vi "PH_Beckhoff_PPMA-Rods.set Digital Input GUI Elements.vi"(2 "Input Up GUI Refs":refnum<vi>[](array[refnum]), 3 "Input GUI Refs":T1, 4 "Digital Inputs":T2, 5 "error in":errorcluster) -> (19 "error out":errorcluster)   [LabVIEW 2014, in "PH_Beckhoff_PPMA-Rods.lvlib"]
doc: "This VI sets the digital Input GUI elements which is whether the rods ar up or not."
uses:
  PH_Beckhoff_PPMA-Rods.lvlib
  PH_Beckhoff/PH_Beckhoff.Digital Inputs.ctl
  PH_Beckhoff_PPMA-Rods.Rods Tags.ctl
  PH_Common/PH_Common.lvlib
  PH_Beckhoff/PH_Beckhoff.lvlib
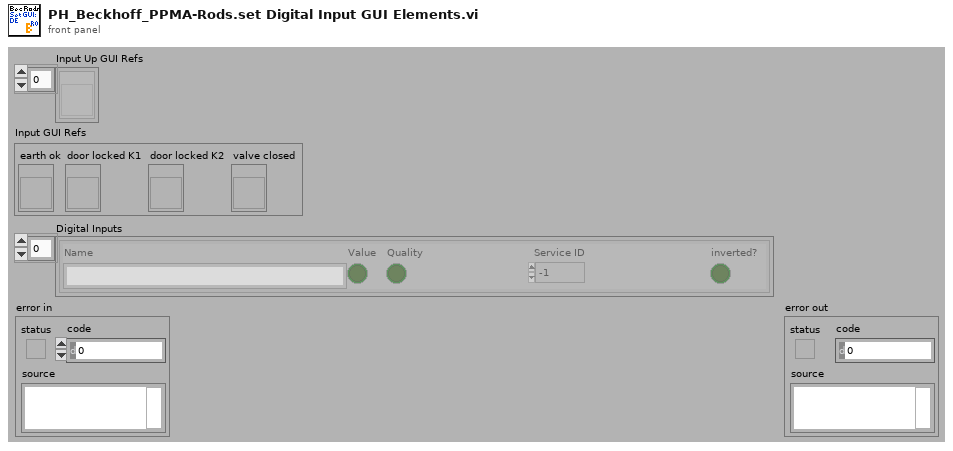
[diagram p1: front panel]
types:
  T1 = cluster{"earth ok":refnum<vi>, "door locked K1":refnum<vi>, "door locked K2":refnum<vi>, "valve closed":refnum<vi>}
  T2 = typedef "PH_Beckhoff.lvlib/PH_Beckhoff.Digital Inputs.ctl" = cluster{"Name":string, "Value":bool, "Quality":bool, "Service ID":i32, "inverted?":bool}[]
  T3 = typedef "PH_Beckhoff_PPMA-Rods.lvlib/PH_Beckhoff_PPMA-Rods.Rods Tags.ctl" = enum16{"Rod-up", "earth-ok", "door-locked-K1", "door-locked-K2", "watervalve-closed", "Rods-Chain-A-up", "Rods-Chain-B-up", "HV-Warnlamp-orange", "HV-Warnlamp-green", "Status-Rods-PU-1", "Status-Rods-PU-2", "Status-Rods-PU-3", "Status-Rods-PU-4", "Status-Rods-PU-5", "Status-Rods-PU-6", "Status-Rods-PU-7", "Status-Rods-PU-8", "Status-Rods-PU-9", "Status-Rods-PU-10", "Status-Rods-FR", "Status-Rods-PILC"}
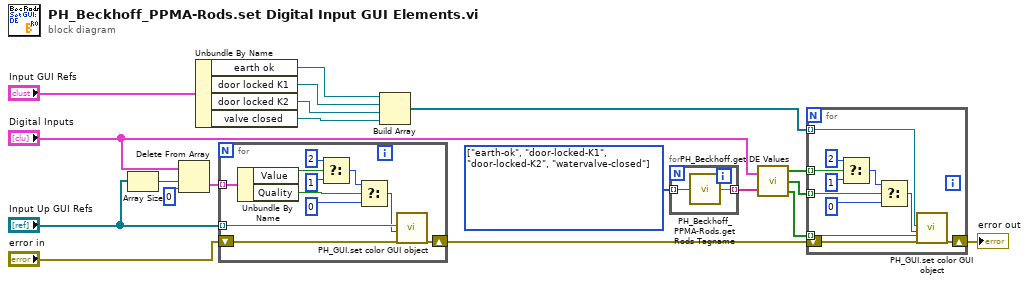
[diagram p0: block diagram]
diagram:
  w7 = T3[] [enum."earth-ok", enum."door-locked-K1", enum."door-locked-K2", enum."watervalve-closed"] items=["Rod-up", "earth-ok", "door-locked-K1", "door-locked-K2", "watervalve-closed", "Rods-Chain-A-up", "Rods-Chain-B-up", "HV-Warnlamp-orange", "HV-Warnlamp-green", "Status-Rods-PU-1", "Status-Rods-PU-2", "Status-Rods-PU-3", "Status-Rods-PU-4", "Status-Rods-PU-5", "Status-Rods-PU-6", "Status-Rods-PU-7", "Status-Rods-PU-8", "Status-Rods-PU-9", "Status-Rods-PU-10", "Status-Rods-FR", "Status-Rods-PILC"]
  n1 = Array Size(array="Input Up GUI Refs") -> (size(s)=w16:i32)
  n2 = Delete From Array(array="Digital Inputs", length=w16, index=0) -> (deleted portion=w1:T2)  [unwired: 1 out]
  n3 = Unbundle By Name("Input GUI Refs") -> ("earth ok"=w9:refnum<vi>, "door locked K1"=w10:refnum<vi>, "door locked K2"=w11:refnum<vi>, "valve closed"=w12:refnum<vi>)
  n4 = for {
    shift-right: [w30] -> w15
    shift-left: "error in" -> [w29]
    tunnel: "Input Up GUI Refs" -> [w28] mode=indexing
    tunnel: w1 -> [w27] mode=indexing
    n5 = Unbundle By Name(w27) -> ("Value"=w23:bool, "Quality"=w26:bool)
    n6 = Select(t=2 ("State"), s=w23, f=1 ("State")) -> (s? t:f=w22:i32)
    n7 = Select(t=w22, s=w26, f=0 ("State")) -> (s? t:f=w24:i32)
    n8 = call "PH_GUI.set color GUI object.vi"("GUI object Ref"=w28, "State"=w24, "error in (no error)"=w29) -> ("error out"=w30:errorcluster)  [unwired: 16 in]
  }
  n9 = Build Array(w9, w10, w11, w12) -> (w8:refnum<vi>[])
  n10 = for {
    tunnel: w7 -> [w32] mode=indexing
    tunnel: [w31] -> w6 mode=indexing
    n11 = call "PH_Beckhoff_PPMA-Rods.get Rods Tagname.vi"("Rods Tag"=w32) -> ("Rods Tagname"=w31:string)
  }
  n12 = call "PH_Beckhoff.get DE Values.vi"("Digital Inputs"="Digital Inputs", "Tags to get"=w6) -> ("Values"=w5:bool[], "Qualities"=w4:bool[], "Tags not found?"=w3:bool[])
  n13 = for {
    shift-right: [w43] -> w14
    shift-left: w15 -> [w42]
    tunnel: w8 -> [w41] mode=indexing
    tunnel: w5 -> [w35] mode=indexing
    tunnel: w4 -> [w34] mode=indexing
    tunnel: w3 -> [w33] mode=indexing
    n14 = Select(t=2 ("State"), s=w35, f=1 ("State")) -> (s? t:f=w38:i32)
    n15 = Select(t=w38, s=w34, f=0 ("State")) -> (s? t:f=w39:i32)
    n16 = call "PH_GUI.set color GUI object.vi"("GUI object Ref"=w41, "State"=w39, "Blinking? (false)"=w33, "error in (no error)"=w42) -> ("error out"=w43:errorcluster)  [unwired: 15 in]
  }
  "error out" <- w14
